vi "SimpleImputer.vi"(8 "error in":errorcluster caption="entrée d'erreur", 11 "SimpleImputer":T1={"missing_values"="nan", "strategy"="mean", "fill_value"={"dtype"="None", "str"="None", "int"=0}, "verbose"=0, "copy"=TRUE, "add_indicator"=FALSE}) -> (0 "error out":errorcluster caption="sortie d'erreur", 3 "SimpleImputer.lvclass":refnum<class "SimpleImputer.lvclass">)   [LabVIEW 2020]
doc: "Imputation transformer for completing missing values.\n\nParameters :\n\n- missing_values : number, string, np.nan (default) or None\nThe placeholder for the missing values. All occurrences of missing_values will be imputed. For pandas’ dataframes with nullable integer dtypes with missing values, missing_values should be set to np.nan, since pd.NA will be converted to np.nan.\n\n- strategy : string, default=’mean’\nThe imputation strategy.\n\nIf “mean”, then replace missing values using the mean along each column. Can only be used with numeric data.\n\nIf “median”, then replace missing values using the median along each column. Can only be used with numeric data.\n\nIf “most_frequent”, then replace missing using the most frequent value along each column. Can be used with strings or numeric data.\n\nIf “constant”, then replace missing values with fill_value. Can be used with strings or numeric data.\n\n- fill_value : string or numerical value, default=None\nWhen strategy == “constant”, fill_value is used to replace all occurrences of missing_values. If left to the default, fill_value will be 0 when imputing numerical data and “missing_value” for strings or object data types.\n\n- verbose : integer, default=0\nControls the verbosity of the imputer.\n\n- copy : boolean, default=True\nIf True, a copy of X will be created. If False, imputation will be done in-place whenever possible. Note that, in the following cases, a new copy will always be made, even if copy=False:\n\nIf X is not an array of floating values;\n\nIf X is encoded as a CSR matrix;\n\nIf add_indicator=True.\n\n- add_indicator : boolean, default=False\nIf True, a MissingIndicator transform will stack onto output of the imputer’s transform. This allows a predictive estimator to account for missingness despite imputation. If a feature has no missing values at fit/train time, the feature won’t appear on the missing indicator even if there are missing values at transform/test time.\n\n\nMethods :\n\n\n- Fit : Fit the imputer on X.\n\nParameters : X : {array-like, sparse matrix}, shape (n_samples, n_features)\n Input data, where n_samples is the number of samples and n_features is the number of features.\n\n\n- Fit Transform : Fit to data, then transform it. Fits transformer to X and y with optional parameters fit_params and returns a transformed version of X.\n\nParameters : X : {array-like, sparse matrix, dataframe} of shape (n_samples, n_features)\n y : ndarray of shape (n_samples,), default=None\n Target values.\n\nReturns : X_new : ndarray array of shape (n_samples, n_features_new)\n Transformed array.\n\n\n- Transform : Impute all missing values in X.\n\nParameters : X : {array-like, sparse matrix}, shape (n_samples, n_features)\n The input data to complete."
uses:
  SimpleImputer.lvclass
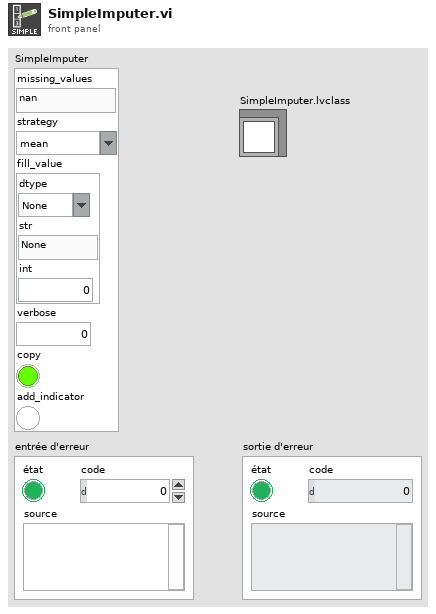
[diagram p1: front panel]
types:
  T1 = cluster{"missing_values":string, "strategy":string, "fill_value":cluster{"dtype":string, "str":string, "int":i32}, "verbose":i32, "copy":bool, "add_indicator":bool}
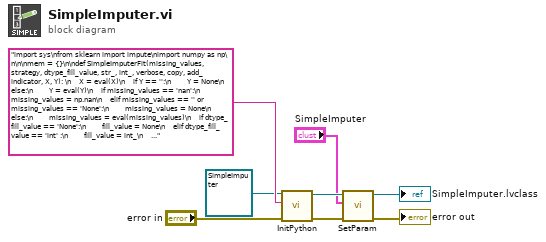
[diagram p0: block diagram]
diagram:
  n1 = call-dynamic "InitPython.vi"("error in (no error)"="error in", "Python Instruction"="import sys\nfrom sklearn import impute\nimport numpy as np\n\n\nmem = {}\n\ndef SimpleImputerFit(missing_values, strategy, dtype_fill_value, str_, int_, verbose, copy, add_indicator, X, Y): \n    X = eval(X)\n    if Y == '':\n        Y = None\n    else:\n        Y = eval(Y)\n    if missing_values == 'nan':\n        missing_values = np.nan\n    elif missing_values == '' or missing_values == 'None':\n        missing_values = None\n    else:\n        missing_values = eval(missing_values)\n    if dtype_fill_value == 'None':\n        fill_value = None\n    elif dtype_fill_value == 'int' :\n        fill_value = int_\n    else:\n        fill_value = str_  \n    try:\n        SimpleImputer = impute.SimpleImputer(missing_values, strategy, fill_value, verbose, copy, add_indicator).fit(X, Y)\n        mem['FitSimpleImputer'] = SimpleImputer\n        return str('OK')\n    except:\n        erreur = sys.exc_info()\n        typerr = u\"%s\" % (erreur[0])\n        typerr = typerr[typerr.find(\"'\")+1:typerr.rfind(\"'\")]\n        msgerr = u\"%s\" % (erreur[1])\n        message = str('/!\\\\ {0} : {1}'. format(typerr,msgerr))\n        return message \n\ndef SimpleImputerFitTransform(missing_values, strategy, dtype_fill_value, str_, int_, verbose, copy, add_indicator, X, Y):\n    X = eval(X)\n    if Y == '':\n        Y = None\n    else:\n        Y = eval(Y)\n    if missing_values == 'nan':\n        missing_values = np.nan\n    elif missing_values == '' or missing_values == 'None':\n        missing_values = None\n    else:\n        missing_values = eval(missing_values)\n    if dtype_fill_value == 'None':\n        fill_value = None\n    elif dtype_fill_value == 'int' :\n        fill_value = int_\n    else:\n        fill_value = str_  \n    try:\n        SimpleImputer = impute.SimpleImputer(missing_values, strategy, fill_value, verbose, copy, add_indicator).fit_transform(X, Y)\n        SimpleImputer = SimpleImputer.tolist()\n        return str(SimpleImputer)\n    except:\n        erreur = sys.exc_info()\n        typerr = u\"%s\" % (erreur[0])\n        typerr = typerr[typerr.find(\"'\")+1:typerr.rfind(\"'\")]\n        msgerr = u\"%s\" % (erreur[1])\n        message = str('/!\\\\ {0} : {1}'. format(typerr,msgerr))\n        return message \n    \n\ndef SimpleImputerTransform(missing_values, strategy, dtype_fill_value, str_, int_, verbose, copy, add_indicator, X, Y): \n    X = eval(X)\n    if Y == '':\n        Y = None\n    else:\n        Y = eval(Y)\n    if missing_values == 'nan':\n        missing_values = np.nan\n    elif missing_values == '' or missing_values == 'None':\n        missing_values = None\n    else:\n        missing_values = eval(missing_values)\n    if dtype_fill_value == 'None':\n        fill_value = None\n    elif dtype_fill_value == 'int' :\n        fill_value = int_\n    else:\n        fill_value = str_  \n    try:\n        SimpleImputer = mem['FitSimpleImputer'].transform(X, Y)\n        SimpleImputer = SimpleImputer.tolist()\n        return str(SimpleImputer)\n    except:\n        erreur = sys.exc_info()\n        typerr = u\"%s\" % (erreur[0])\n        typerr = typerr[typerr.find(\"'\")+1:typerr.rfind(\"'\")]\n        msgerr = u\"%s\" % (erreur[1])\n        message = str('/!\\\\ {0} : {1}'. format(typerr,msgerr))\n        return message", "Scikit-learn en entrée"=refnum<class "SimpleImputer.lvclass"> refnum ("SimpleImputer.lvclass")) -> ("error out"=w4:errorcluster, "Scikit-learn en sortie"=w5:refnum<class "SimpleImputer.lvclass">)  [unwired: 7 in]
  n2 = call-dynamic "SetParam.vi"("error in (no error)"=w4, "SimpleImputer"="SimpleImputer", "SimpleImputer.lvclass"=w5) -> ("error out"=→"error out":errorcluster, "SimpleImputer.lvclass"=→"SimpleImputer.lvclass":refnum<class "SimpleImputer.lvclass">)  [unwired: 7 in]
